vi "SensorDataUpdater.vi"() -> ()   [LabVIEW 2012]
uses:
  BotStatus.vi
panel:
  in  "reset":bool
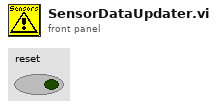
[diagram p1: front panel]
types:
  T1 = typedef "WPI_AnalogChannelDevRef.ctl" = cluster{"DevStatus":errorcluster, "Analog Module":T2, "Analog Channel":T3}
  T2 = typedef "FPGA_TypedefAnalogModule.ctl" = enum16{"Analog Module 1", "Analog Module 2"}
  T3 = typedef "FPGA_AIChannel.ctl" = enum8{"AI 1", "AI 2", "AI 3", "AI 4", "AI 5", "AI 6", "AI 7", "AI 8", "Invalid"}
  T4 = typedef "WPI_DigitalInputDevRef.ctl" = cluster{"DevStatus":errorcluster, "DIO Channel":T5, "Digital Module":T6}
  T5 = typedef "FPGA_DIOChannel.ctl" = enum8{"DIO 1", "DIO 2", "DIO 3", "DIO 4", "DIO 5", "DIO 6", "DIO 7", "DIO 8", "DIO 9", "DIO 10", "DIO 11", "DIO 12", "DIO 13", "DIO 14", "Invalid"}
  T6 = typedef "FPGA_TypedefDigitalModule.ctl" = enum16{"Digital Module 1", "Digital Module 2"}
  T7 = typedef "WPI_ServoDeviceRef.ctl" = cluster{"DeviceStatus":errorcluster, "Digital Module":T6, "PWM Channel":T8, "DeadBand":T9}
  T8 = typedef "FPGA_DIOPWMChannel.ctl" = enum8{"PWM 1", "PWM 2", "PWM 3", "PWM 4", "PWM 5", "PWM 6", "PWM 7", "PWM 8", "PWM 9", "PWM 10", "Invalid"}
  T9 = typedef "WPI_PWMDeadband.ctl" = cluster{"Name":string, "maxPositivePwm":i32, "minPositivePwm":i32, "centerPwm":i32, "maxNegativePwm":i32, "minNegativePwm":i32, "angularRange":u16}
  T10 = cluster{"Middle":bool, "InCannon":bool, "InFlipper":bool, "FlipperAtPlace":bool, "Bottom":bool, "FrisbeeDirection":bool}
  T11 = cluster{"Cannon Upper LS":bool, "Cannon Lower LS":bool}
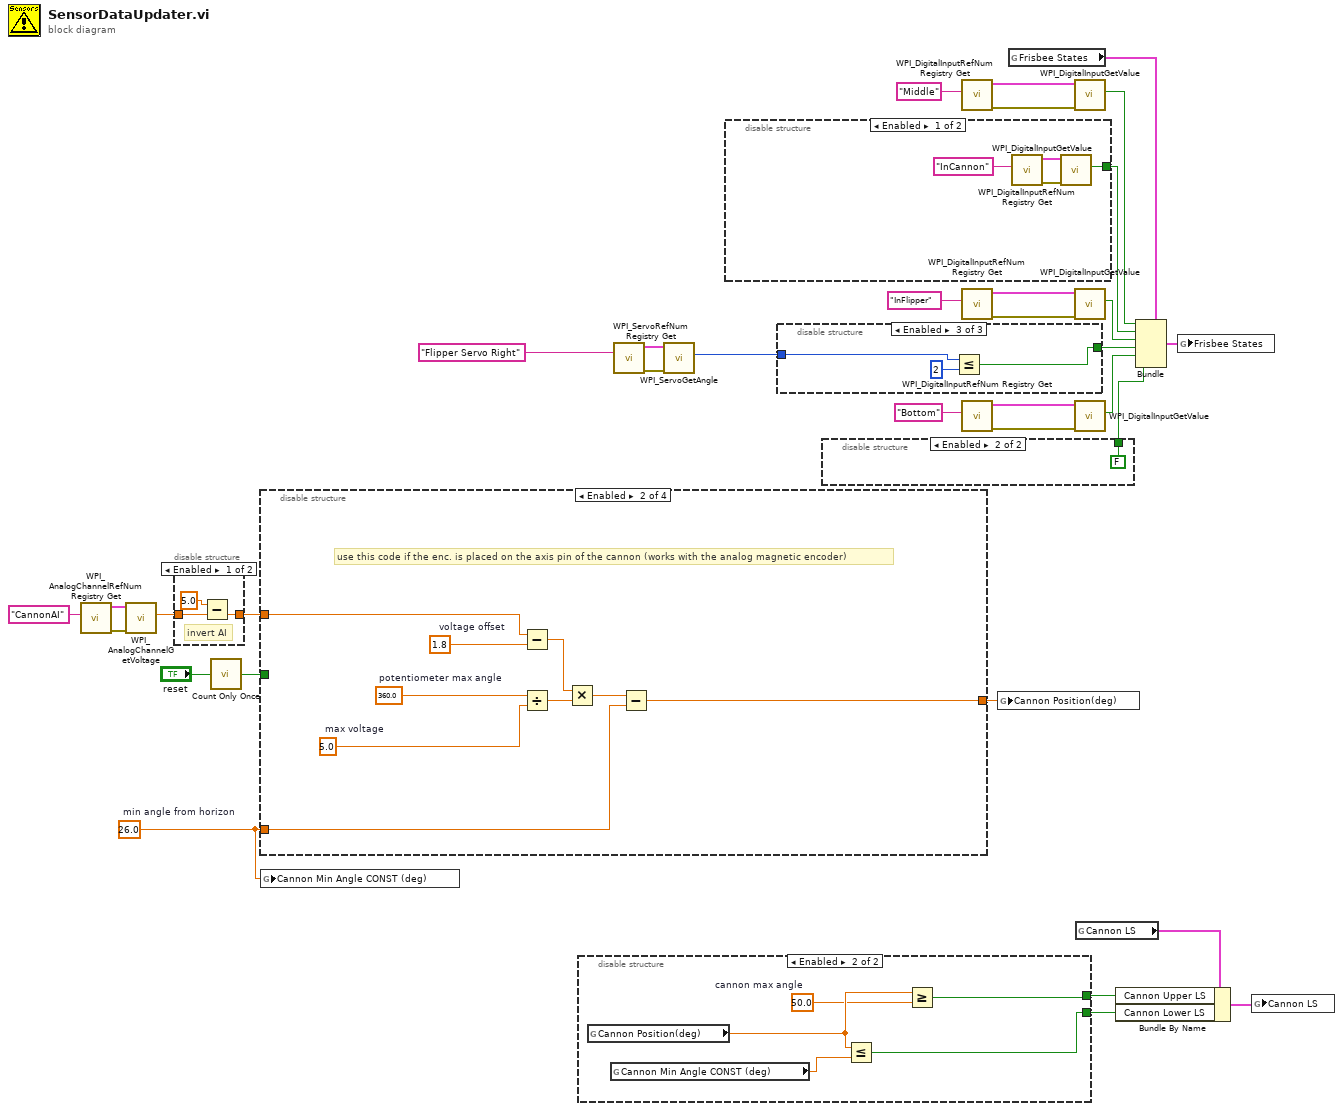
[diagram p0: block diagram]
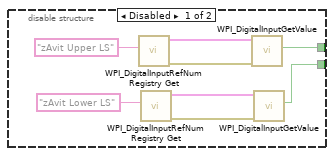
[diagram p2: hidden frame]
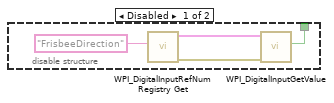
[diagram p3: hidden frame]
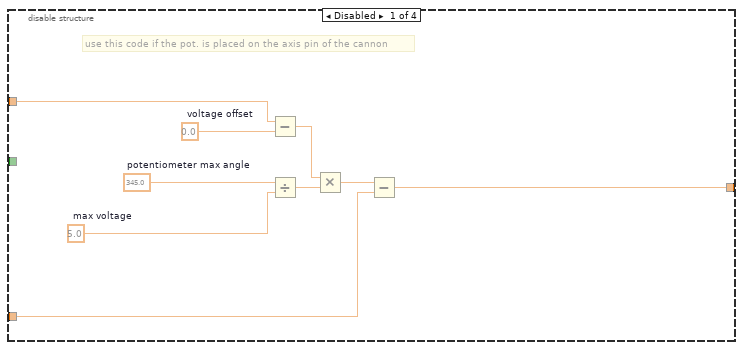
[diagram p5: hidden frame]
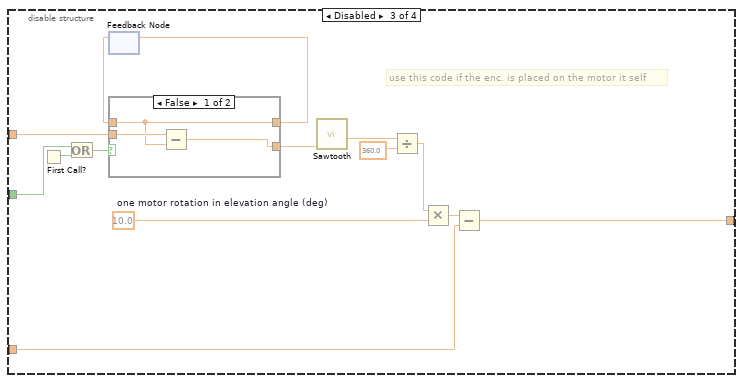
[diagram p6: hidden frame]
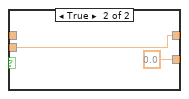
[diagram p7: hidden frame]
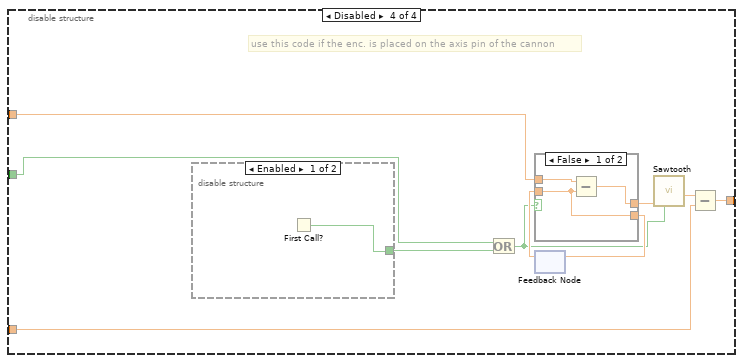
[diagram p8: hidden frame]
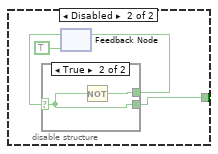
[diagram p9: hidden frame]
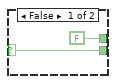
[diagram p10: hidden frame]
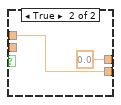
[diagram p11: hidden frame]
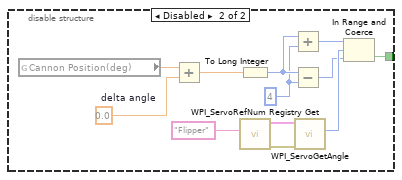
[diagram p12: hidden frame]
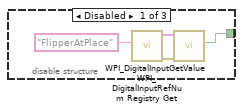
[diagram p13: hidden frame]
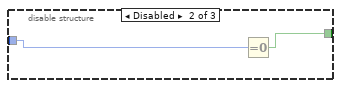
[diagram p14: hidden frame]
diagram:
  w12 = 26.0  # min angle from horizon
  n1 = call <vilib>:"WPI_AnalogChannelRefNum Registry Get.vi"("refnum name"="CannonAI") -> ("error out"=w14:errorcluster, "AIDeviceRef"=w16:T1)  [unwired: 9 in]
  n2 = call <vilib>:"WPI_AnalogChannelGetVoltage.vi"("error in (no error)"=w14, "AIDeviceRef"=w16) -> ("Voltage"=w15:dbl)  [unwired: 7 in, 2 out]
  n3 = disable-structure shown="Enabled" {
    disable-tunnel: w15 -> [w37 w38]
    disable-tunnel: [w36 w38] -> w5
    frame Enabled {
      # "invert AI"
      n4 = Subtract(x=5.0, y=w37) -> (x-y=w36:dbl)
    }
    frame Disabled {
    }
  }
  n5 = call "Count Only Once.vi"("InValue"="reset") -> ("Result"=w6:bool)
  n6 = disable-structure shown="Enabled" {
    disable-tunnel: w5 -> [w47 w56 w63 w83]
    disable-tunnel: [w42 w51 w69 w84] -> w13
    disable-tunnel: w12 -> [w39 w48 w70 w85]
    disable-tunnel: w6 -> [_ _ w58 w78]
    frame Disabled {
      w40 = 0.0  # voltage offset
      w44 = 5.0  # max voltage
      w45 = 345.0  # potentiometer max angle
      # "use this code if the pot. is placed on the axis pin of the cannon"
      n7 = Subtract(x=w47, y=w40) -> (x-y=w41:dbl)
      n8 = Divide(x=w45, y=w44) -> (x/y=w43:dbl)
      n9 = Multiply(x=w41, y=w43) -> (x*y=w46:dbl)
      n10 = Subtract(x=w46, y=w39) -> (x-y=w42:dbl)
    }
    frame Enabled {
      w49 = 1.8  # voltage offset
      w53 = 5.0  # max voltage
      w54 = 360.0  # potentiometer max angle
      # "use this code if the enc. is placed on the axis pin of the cannon (works with the analog magnetic encoder)"
      n11 = Subtract(x=w56, y=w49) -> (x-y=w50:dbl)
      n12 = Divide(x=w54, y=w53) -> (x/y=w52:dbl)
      n13 = Multiply(x=w50, y=w52) -> (x*y=w55:dbl)
      n14 = Subtract(x=w55, y=w48) -> (x-y=w51:dbl)
    }
    frame Disabled {
      w64 = 10.0  # one motor rotation in elevation angle (deg)
      # "use this code if the enc. is placed on the motor it self"
      n15 = First Call?() -> (First Call?: T/F=w59:bool)
      n16 = Or(x=w58, y=w59) -> (x .or. y?=w57:bool)
      n17 = feedback #1() -> (w61:dbl)  [unwired: 1 in]
      n18 = case shown="False" w57 {
        tunnel: w63 -> [w73 w75]
        tunnel: [w72 w75] -> w62
        tunnel: w61 -> [w72 _]
        tunnel: [w71 0.0] -> w60
        frame False {
          n19 = Subtract(x=w73, y=w72) -> (x-y=w71:dbl)
        }
        frame True {
        }
      }
      n20 = feedback-in #1(w62) -> ()
      n21 = call "Sawtooth.vi"("Voltage"=w60) -> ("Absolute Angle (deg)"=w68:dbl)  [unwired: 8 in, 2 out]
      n22 = Divide(x=w68, y=360.0) -> (x/y=w66:dbl)
      n23 = Multiply(x=w66, y=w64) -> (x*y=w65:dbl)
      n24 = Subtract(x=w65, y=w70) -> (x-y=w69:dbl)
    }
    frame Disabled {
      # "use this code if the enc. is placed on the axis pin of the cannon"
      n25 = disable-structure shown="Enabled" {
        disable-tunnel: [w86 w88] -> w79
        frame Enabled {
          n26 = First Call?() -> (First Call?: T/F=w86:bool)
        }
        frame Disabled {
          n27 = feedback #2(TRUE) -> (w90:bool)
          n28 = case shown="True" w90 {
            selector: w90 -> [w92 w94]
            tunnel: [w92 w94] -> w88
            tunnel: [FALSE w93] -> w87
            frame False {
            }
            frame True {
              n29 = Not(x=w94) -> (.not. x?=w93:bool)
            }
          }
          n30 = feedback-in #2(w87) -> ()
        }
      }
      n31 = Or(x=w78, y=w79) -> (x .or. y?=w76:bool)
      n32 = feedback #3() -> (w81:dbl)  [unwired: 1 in]
      n33 = case shown="False" w76 {
        tunnel: w83 -> [w97 w99]
        tunnel: [w96 w99] -> w82
        tunnel: w81 -> [w96 _]
        tunnel: [w95 0.0] -> w80
        frame False {
          n34 = Subtract(x=w97, y=w96) -> (x-y=w95:dbl)
        }
        frame True {
        }
      }
      n35 = feedback-in #3(w82) -> ()
      n36 = call "Sawtooth.vi"("Reintalize?"=w76, "Voltage"=w80) -> ("Absolute Angle (deg)"=w77:dbl)  [unwired: 7 in, 2 out]
      n37 = Subtract(x=w77, y=w85) -> (x-y=w84:dbl)
    }
  }
  n38 = global write "BotStatus.vi" "Cannon Min Angle CONST (deg)"(w12) -> ()
  n39 = disable-structure shown="Enabled" {
    disable-tunnel: [w104 w108] -> w2
    disable-tunnel: [w100 w111] -> w1
    frame Disabled {
      n40 = call <vilib>:"WPI_DigitalInputRefNum Registry Get.vi"("refnum name"="zAvit Upper LS") -> ("error out"=w106:errorcluster, "DigitalInputDevRef"=w107:T4)  [unwired: 9 in]
      n41 = call <vilib>:"WPI_DigitalInputRefNum Registry Get.vi"("refnum name"="zAvit Lower LS") -> ("error out"=w102:errorcluster, "DigitalInputDevRef"=w101:T4)  [unwired: 9 in]
      n42 = call <vilib>:"WPI_DigitalInputGetValue.vi"("error in (no error)"=w106, "DigitalInputDevRef"=w107) -> ("Value"=w104:bool)  [unwired: 7 in, 2 out]
      n43 = call <vilib>:"WPI_DigitalInputGetValue.vi"("error in (no error)"=w102, "DigitalInputDevRef"=w101) -> ("Value"=w100:bool)  [unwired: 7 in, 2 out]
    }
    frame Enabled {
      w109 = 50.0  # cannon max angle
      n44 = global read "BotStatus.vi" "Cannon Position(deg)"() -> (w110:dbl)
      n45 = global read "BotStatus.vi" "Cannon Min Angle CONST (deg)"() -> (w112:dbl)
      n46 = Less Or Equal?(x=w110, y=w112) -> (x <= y?=w111:bool)
      n47 = Greater Or Equal?(x=w110, y=w109) -> (x >= y?=w108:bool)
    }
  }
  n48 = call <vilib>:"WPI_ServoRefNum Registry Get.vi"("refnum name"="Flipper Servo Right") -> ("error out"=w11:errorcluster, "ServoDeviceRef"=w10:T7)  [unwired: 9 in]
  n49 = call <vilib>:"WPI_ServoGetAngle.vi"("ServoDeviceRef"=w10, "error in (no error)"=w11) -> ("Angle"=w8:u16)  [unwired: 6 in, 2 out]
  n50 = disable-structure shown="Enabled" {
    disable-tunnel: [w113 w117] -> w21
    frame Enabled {
      n51 = call <vilib>:"WPI_DigitalInputRefNum Registry Get.vi"("refnum name"="InCannon") -> ("error out"=w115:errorcluster, "DigitalInputDevRef"=w114:T4)  [unwired: 9 in]
      n52 = call <vilib>:"WPI_DigitalInputGetValue.vi"("error in (no error)"=w115, "DigitalInputDevRef"=w114) -> ("Value"=w113:bool)  [unwired: 7 in, 2 out]
    }
    frame Disabled {
      w119 = 4 ("y")
      w124 = 0.0  # delta angle
      n53 = global read "BotStatus.vi" "Cannon Position(deg)"() -> (w125:dbl)
      n54 = Add(x=w125, y=w124) -> (x+y=w123:dbl)
      n55 = To Long Integer(number=w123) -> (32bit integer=w120:i32)
      n56 = call <vilib>:"WPI_ServoRefNum Registry Get.vi"("refnum name"="Flipper") -> ("error out"=w128:errorcluster, "ServoDeviceRef"=w127:T7)  [unwired: 9 in]
      n57 = Add(x=w120, y=w119) -> (x+y=w121:i32)
      n58 = Subtract(x=w120, y=w119) -> (x-y=w118:i32)
      n59 = call <vilib>:"WPI_ServoGetAngle.vi"("ServoDeviceRef"=w127, "error in (no error)"=w128) -> ("Angle"=w122:u16)  [unwired: 6 in, 2 out]
      n60 = In Range and Coerce(upper limit=w121, x=w122, lower limit=w118) -> (In Range?=w117:bool)  [unwired: 1 out]
    }
  }
  n61 = disable-structure shown="Enabled" {
    disable-tunnel: [w129 w134 w136] -> w19
    disable-tunnel: w8 -> [_ w133 w135]
    frame Disabled {
      n62 = call <vilib>:"WPI_DigitalInputRefNum Registry Get.vi"("refnum name"="FlipperAtPlace") -> ("error out"=w131:errorcluster, "DigitalInputDevRef"=w132:T4)  [unwired: 9 in]
      n63 = call <vilib>:"WPI_DigitalInputGetValue.vi"("error in (no error)"=w131, "DigitalInputDevRef"=w132) -> ("Value"=w129:bool)  [unwired: 7 in, 2 out]
    }
    frame Disabled {
      n64 = Equal To 0?(x=w133) -> (x = 0?=w134:bool)
    }
    frame Enabled {
      n65 = Less Or Equal?(x=w135, y=2) -> (x <= y?=w136:bool)
    }
  }
  n66 = disable-structure shown="Enabled" {
    disable-tunnel: [w138 FALSE ("Value")] -> w18
    frame Disabled {
      n67 = call <vilib>:"WPI_DigitalInputRefNum Registry Get.vi"("refnum name"="FrisbeeDirection") -> ("error out"=w140:errorcluster, "DigitalInputDevRef"=w139:T4)  [unwired: 9 in]
      n68 = call <vilib>:"WPI_DigitalInputGetValue.vi"("error in (no error)"=w140, "DigitalInputDevRef"=w139) -> ("Value"=w138:bool)  [unwired: 7 in, 2 out]
    }
    frame Enabled {
    }
  }
  n69 = call <vilib>:"WPI_DigitalInputRefNum Registry Get.vi"("refnum name"="Middle") -> ("error out"=w26:errorcluster, "DigitalInputDevRef"=w27:T4)  [unwired: 9 in]
  n70 = call <vilib>:"WPI_DigitalInputRefNum Registry Get.vi"("refnum name"="InFlipper") -> ("error out"=w29:errorcluster, "DigitalInputDevRef"=w28:T4)  [unwired: 9 in]
  n71 = call <vilib>:"WPI_DigitalInputRefNum Registry Get.vi"("refnum name"="Bottom") -> ("error out"=w31:errorcluster, "DigitalInputDevRef"=w30:T4)  [unwired: 9 in]
  n72 = global write "BotStatus.vi" "Cannon Position(deg)"(w13) -> ()
  n73 = global read "BotStatus.vi" "Frisbee States"() -> (w25:T10)
  n74 = call <vilib>:"WPI_DigitalInputGetValue.vi"("error in (no error)"=w26, "DigitalInputDevRef"=w27) -> ("Value"=w22:bool)  [unwired: 7 in, 2 out]
  n75 = call <vilib>:"WPI_DigitalInputGetValue.vi"("error in (no error)"=w29, "DigitalInputDevRef"=w28) -> ("Value"=w20:bool)  [unwired: 7 in, 2 out]
  n76 = call <vilib>:"WPI_DigitalInputGetValue.vi"("error in (no error)"=w31, "DigitalInputDevRef"=w30) -> ("Value"=w23:bool)  [unwired: 7 in, 2 out]
  n77 = global read "BotStatus.vi" "Cannon LS"() -> (w4:T11)
  n78 = Bundle By Name(cluster=w4, "Cannon Upper LS"=w2, "Cannon Lower LS"=w1) -> (w3:T11)
  n79 = Bundle(cluster=w25, "Middle"=w22, "InCannon"=w21, "InFlipper"=w20, "FlipperAtPlace"=w19, "Bottom"=w23, "FrisbeeDirection"=w18) -> (w24:T10)
  n80 = global write "BotStatus.vi" "Frisbee States"(w24) -> ()
  n81 = global write "BotStatus.vi" "Cannon LS"(w3) -> ()
